vi "CRYRepresent numeric by precission.vi"(10 "Pprecision":u8=2, 11 "Numeric In":dbl format="%#.6p") -> (0 "Out Format":string, 2 "output string":string, 3 "Numeric Out":dbl format="%#.1p")   [LabVIEW 2013]
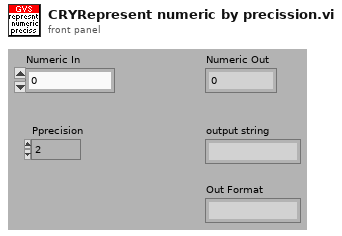
[diagram p1: front panel]
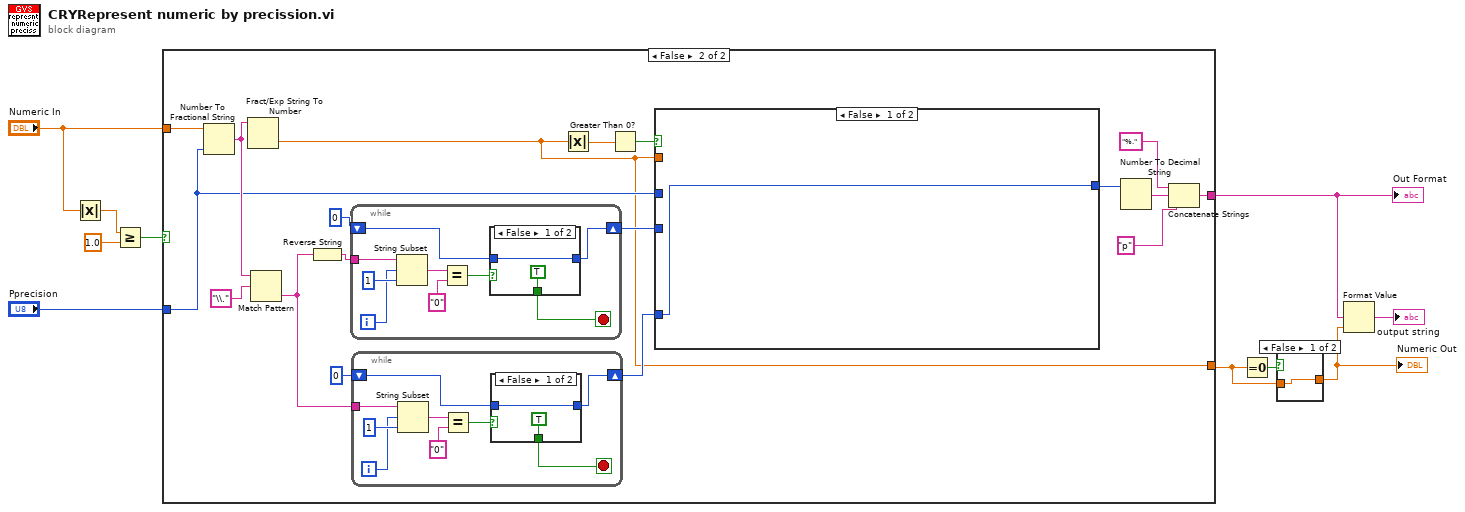
[diagram p0: block diagram]
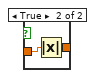
[diagram p2: hidden frame]
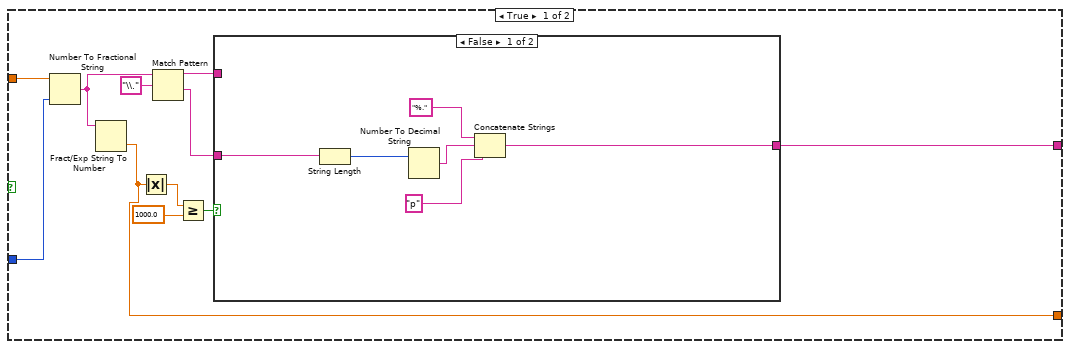
[diagram p3: hidden frame]
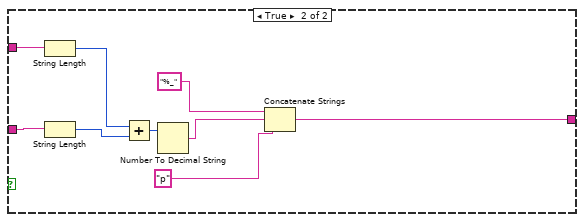
[diagram p4: hidden frame]
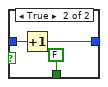
[diagram p5: hidden frame]
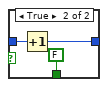
[diagram p6: hidden frame]
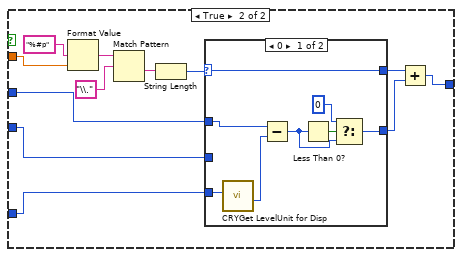
[diagram p7: hidden frame]
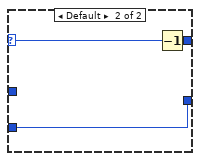
[diagram p8: hidden frame]
diagram:
  n1 = Absolute Value(x="Numeric In") -> (abs(x)=w9:dbl)
  n2 = Greater Or Equal?(x=w9, y=1.0 ("x")) -> (x >= y?=w5:bool)
  n3 = case shown="False" w5 {
    tunnel: "Numeric In" -> [w21 w39]
    tunnel: "Pprecision" -> [w20 w50]
    tunnel: [w12 w42] -> w7
    tunnel: [w11 w37] -> w2
    frame True {
      n4 = Number To Fractional String(number=w21, precision (6)=w20) -> (F-format string=w18:string)  [unwired: 2 in]
      n5 = Fract/Exp String To Number(string=w18) -> (number=w11:dbl)  [unwired: 3 in, 1 out]
      n6 = Absolute Value(x=w11) -> (abs(x)=w15:dbl)
      n7 = Match Pattern(string=w18, regular expression="\\." ("f")) -> (before substring=w13:string, after substring=w14:string)  [unwired: 1 in, 2 out]
      n8 = Greater Or Equal?(x=w15, y=1000.0 ("x")) -> (x >= y?=w16:bool)
      n9 = case shown="False" w16 {
        tunnel: w14 -> [w24 w35]
        tunnel: [w23 w28] -> w12
        tunnel: w13 -> [_ w36]
        frame False {
          n10 = String Length(string=w24) -> (length=w22:i32)
          n11 = Number To Decimal String(number=w22) -> (decimal integer string=w26:string)  [unwired: 1 in]
          n12 = Concatenate Strings("%." ("string"), w26, "p" ("format string")) -> (w23:string)
        }
        frame True {
          n13 = String Length(string=w36) -> (length=w33:i32)
          n14 = String Length(string=w35) -> (length=w34:i32)
          n15 = Add(x=w33, y=w34) -> (x+y=w32:i32)
          n16 = Number To Decimal String(number=w32) -> (decimal integer string=w29:string)  [unwired: 1 in]
          n17 = Concatenate Strings("%_" ("string"), w29, "p" ("format string")) -> (w28:string)
        }
      }
    }
    frame False {
      n18 = Number To Fractional String(number=w39, precision (6)=w50) -> (F-format string=w53:string)  [unwired: 2 in]
      n19 = Fract/Exp String To Number(string=w53) -> (number=w37:dbl)  [unwired: 3 in, 1 out]
      n20 = Match Pattern(string=w53, regular expression="\\." ("f")) -> (after substring=w41:string)  [unwired: 1 in, 3 out]
      n21 = Reverse String(1:w41) -> (0:w44:string)
      n22 = while {
        tunnel: w44 -> [w59]
        shift-right: [w57] -> w43
        shift-left: 0 ("length (rest)") -> [w56]
        i -> [w60]
        stop <- w55 stop-if-true
        n23 = String Subset(string=w59, offset (0)=w60, length (rest)=1 ("length (rest)")) -> (substring=w62:string)
        n24 = Equal?(x=w62, y="0") -> (x = y?=w58:bool)
        n25 = case shown="False" w58 {
          tunnel: w56 -> [w65 w68]
          tunnel: [w65 w67] -> w57
          tunnel: [TRUE FALSE] -> w55
          frame False {
          }
          frame True {
            n26 = Increment(x=w68) -> (x+1=w67:i32)
          }
        }
      }
      n27 = while {
        tunnel: w41 -> [w73]
        shift-right: [w71] -> w49
        shift-left: 0 ("length (rest)") -> [w70]
        i -> [w74]
        stop <- w69 stop-if-true
        n28 = String Subset(string=w73, offset (0)=w74, length (rest)=1 ("length (rest)")) -> (substring=w76:string)
        n29 = Equal?(x=w76, y="0") -> (x = y?=w72:bool)
        n30 = case shown="False" w72 {
          tunnel: w70 -> [w79 w82]
          tunnel: [w79 w81] -> w71
          tunnel: [TRUE FALSE] -> w69
          frame False {
          }
          frame True {
            n31 = Increment(x=w82) -> (x+1=w81:i32)
          }
        }
      }
      n32 = Absolute Value(x=w37) -> (abs(x)=w38:dbl)
      n33 = Greater Than 0?(x=w38) -> (x > 0?=w52:bool)
      n34 = case shown="False" w52 {
        tunnel: w50 -> [_ w87]
        tunnel: w49 -> [w83 w85]
        tunnel: [w83 w91] -> w40
        tunnel: w43 -> [_ w86]
        tunnel: w37 -> [_ w95]
        frame False {
        }
        frame True {
          n35 = Format Value(format string="%#p" ("string (\"\")"), value (0)=w95) -> (output string=w93:string)  [unwired: 1 out]
          n36 = Match Pattern(string=w93, regular expression="\\." ("f")) -> (after substring=w92:string)  [unwired: 1 in, 3 out]
          n37 = String Length(string=w92) -> (length=w89:i32)
          n38 = case shown="0" w89 {
            selector: w89 -> [w103 w106]
            tunnel: [w103 w105] -> w88
            tunnel: w87 -> [w98 _]
            tunnel: w86 -> [_ w104]
            tunnel: w85 -> [w99 _]
            tunnel: [w100 w104] -> w84
            frame 0 {
              n39 = call "CRYGet LevelUnit for Disp.vi"("In Value"=w99) -> ("Lvl Unit"=w97:i16)  [unwired: 10 in]
              n40 = Subtract(x=w98, y=w97) -> (x-y=w96:i16)
              n41 = Less Than 0?(x=w96) -> (x < 0?=w102:bool)
              n42 = Select(t=i16 0 ("y"), s=w102, f=w96) -> (s? t:f=w100:i16)
            }
            frame Default {
              n43 = Decrement(x=w106) -> (x-1=w105:i32)
            }
          }
          n44 = Add(x=w88, y=w84) -> (x+y=w91:i32)
        }
      }
      n45 = Number To Decimal String(number=w40) -> (decimal integer string=w48:string)  [unwired: 1 in]
      n46 = Concatenate Strings("%." ("string"), w48, "p" ("format string")) -> (w42:string)
    }
  }
  "Out Format" <- w7
  n47 = Equal To 0?(x=w2) -> (x = 0?=w3:bool)
  n48 = case shown="False" w3 {
    tunnel: w2 -> [w107 w109]
    tunnel: [w107 w108] -> w1
    frame False {
    }
    frame True {
      n49 = Absolute Value(x=w109) -> (abs(x)=w108:dbl)
    }
  }
  "Numeric Out" <- w1
  n50 = Format Value(format string=w7, value (0)=w1) -> (output string=→"output string":string)  [unwired: 1 out]
